vi "Clear.vi"(8 "error in (no error)":errorcluster, 11 "Pointer in":refnum<class "Pointer.lvclass">) -> (0 "error out":errorcluster, 3 "Pointer out":refnum<class "Pointer.lvclass">)   [LabVIEW 2016, in "Memory Manager.lvlib" / "Pointer.lvclass"]
doc: "Sets all of the bytes specified by <b>pointer</b> to zero.\n\n<b>Note:</b> This VI is <b>safe</b>, meaning it performs null pointer and bounds checks to prevent invaid memory access."
uses:
  Pointer.lvclass
  Pointer.lvclass/Pointer.ctl
  Errors.vi
  Null Pointer.vi
  Get Address.vi
  Clear Subset (No Check).vi
  Create Error.vi
  Get Size.vi
  Get Error Info.vi
  VIs/Source.Write.String.vi
  VIs/Error Cluster.Set VI Source.vi
  VIs/Error Cluster.Set Code.vi
  VIs/Error Cluster.Set Status.vi
  VIs/New Error Cluster Constant.vi
  VIs/New Error Cluster Constant (512B).vi
  Constants/Constants.vi
  Constants/Library Name.vi
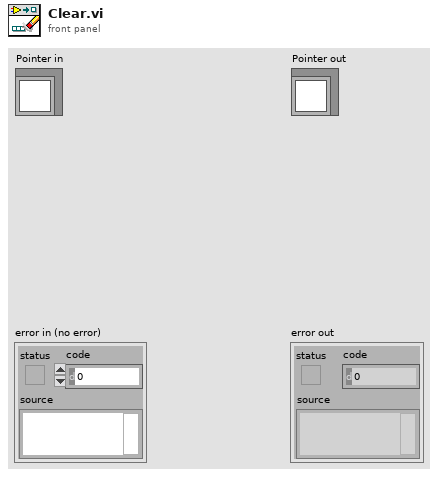
[diagram p1: front panel]
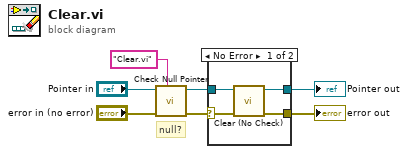
[diagram p0: block diagram]
diagram:
  # "null?"
  n1 = call "Check Null Pointer.vi"("source vi name"="Clear.vi", "error in (no error)"="error in (no error)", "Pointer in"="Pointer in") -> ("error out"=w1:errorcluster, "Pointer out"=w4:refnum<class "Pointer.lvclass">)  [unwired: 7 in]
  n2 = case shown="No Error" w1 {
    selector: w1 -> [w8 w13]
    tunnel: w4 -> [w11 w12]
    tunnel: [w10 w12] -> w3
    tunnel: [w9 w13] -> w2
    frame No Error {
      n3 = call "Clear (No Check).vi"("error in (no error)"=w8, "Pointer in"=w11) -> ("error out"=w9:errorcluster, "Pointer out"=w10:refnum<class "Pointer.lvclass">)  [unwired: 8 in]
    }
    frame Error {
    }
  }
  "error out" <- w2
  "Pointer out" <- w3
